vi "ep_Compute Third Current (Spectra).vi"(0 "complex current spectra in (5Hz step)":T2(array[cluster]), 5 "wiring":T3, 11 "error in (no error)":errorcluster) -> (4 "complex current spectra out (5Hz step)":T2(array[cluster]), 15 "error out":errorcluster)   [LabVIEW 2011, in "NI_EP_Power Quality.lvlib"]
uses:
  <vilib>/addons/Electrical Power/PQ/NI_EP_Power Quality.lvlib
  <vilib>/addons/Electrical Power/PQ/Common/Controls/ep_AI Data Channel.ctl
  <vilib>/addons/Electrical Power/PQ/Common/Controls/ep_Wiring.ctl
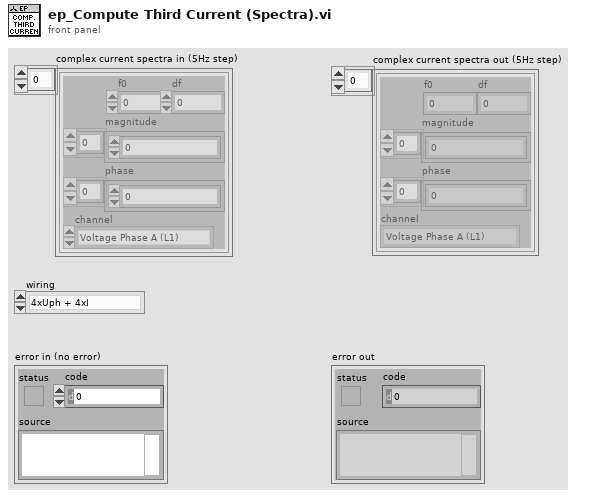
[diagram p1: front panel]
types:
  T1 = typedef "NI_EP_Power Quality.lvlib/ep_AI Data Channel.ctl" = enum16{"Voltage Phase A (L1)", "Voltage Phase B (L2)", "Voltage Phase C (L3)", "Voltage Phase N (Neutral)", "Current Phase A (L1)", "Current Phase B (L2)", "Current Phase C (L3)", "Current Phase N (Neutral)"}
  T2 = cluster{"f0":dbl, "df":dbl, "magnitude":dbl[], "phase":dbl[], "channel":T1}[]
  T3 = typedef "NI_EP_Power Quality.lvlib/ep_Wiring.ctl" = enum16{"4xUph + 4xI", "3xUph + 4xI", "3xUline + 4xI", "3xUph + 3xI", "3xUline + 3xI", "3xUph + 2xI", "3xUline + 2xI", "1xUph + 1xI"}
  T4 = cluster{"f0":dbl, "df":dbl, "magnitude":dbl[], "phase":dbl[], "channel":T1}
  T5 = cluster{"f0":dbl, "df":dbl, dbl[], dbl[], "AI data channel":T1}
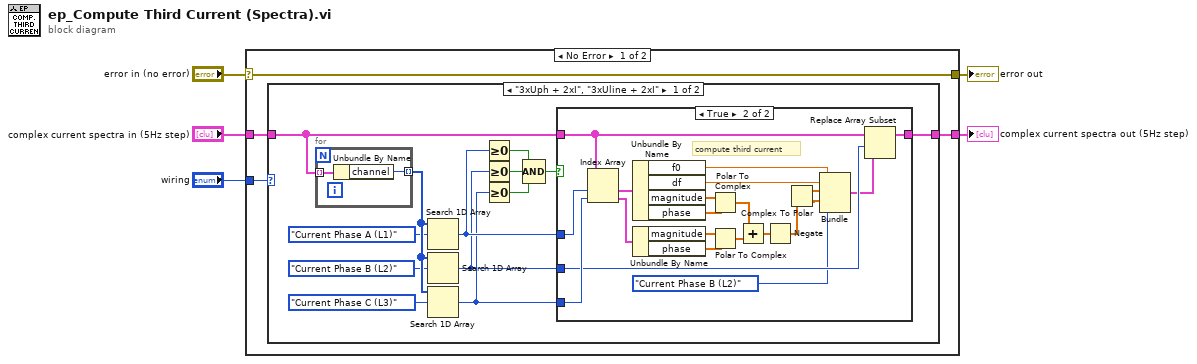
[diagram p0: block diagram]
diagram:
  n1 = case shown="No Error" "error in (no error)" {
    selector: "error in (no error)" -> [w6 w48]
    tunnel: "wiring" -> [w9 _]
    tunnel: [w8 _] -> w4
    tunnel: "complex current spectra in (5Hz step)" -> [w7 _]
    tunnel: [w6 w48] -> w1
    frame No Error {
      n2 = case shown="\"3xUph + 2xI\", \"3xUline + 2xI\"" w9 {
        tunnel: w7 -> [w11 w47]
        tunnel: [w22 w47] -> w8
        frame "3xUph + 2xI", "3xUline + 2xI" {
          n3 = for {
            tunnel: w11 -> [w46] mode=indexing
            tunnel: [w45] -> w19 mode=indexing
            n4 = Unbundle By Name(w46) -> ("channel"=w45:T1)
          }
          n5 = Search 1D Array(1D array=w19, element=ep_AI_Data_Channel."Current Phase A (L1)" ("AI data channel")) -> (index of element=w14:i32)  [unwired: 1 in]
          n6 = Search 1D Array(1D array=w19, element=ep_AI_Data_Channel."Current Phase B (L2)" ("AI data channel")) -> (index of element=w12:i32)  [unwired: 1 in]
          n7 = Search 1D Array(1D array=w19, element=ep_AI_Data_Channel."Current Phase C (L3)" ("AI data channel")) -> (index of element=w13:i32)  [unwired: 1 in]
          n8 = Greater Or Equal To 0?(x=w14) -> (x >= 0?=w10:bool)
          n9 = Greater Or Equal To 0?(x=w12) -> (x >= 0?=w20:bool)
          n10 = Greater Or Equal To 0?(x=w13) -> (x >= 0?=w21:bool)
          n11 = Compound Arithmetic op=AND(w10, w20, w21) -> (w15:bool)
          n12 = case shown="True" w15 {
            tunnel: [w23 w44] -> w22
            tunnel: w11 -> [w23 w43]
            tunnel: w14 -> [_ w42]
            tunnel: w13 -> [_ w41]
            tunnel: w12 -> [_ w40]
            frame False {
            }
            frame True {
              # "compute third current"
              n13 = Index Array(array=w43, index #1=w42, index #2=w41) -> (element #1=w39:T4, element #2=w38:T4)
              n14 = Unbundle By Name(w39) -> ("f0"=w36:dbl, "df"=w34:dbl, "magnitude"=w33:dbl[], "phase"=w32:dbl[])
              n15 = Unbundle By Name(w38) -> ("magnitude"=w30:dbl[], "phase"=w29:dbl[])
              n16 = Polar To Complex(1:w32, 2:w33) -> (0:w31:cdb[])
              n17 = Polar To Complex(1:w29, 2:w30) -> (0:w28:cdb[])
              n18 = Add(x=w31, y=w28) -> (x+y=w37:cdb[])
              n19 = Negate(x=w37) -> (-x=w24:cdb[])
              n20 = Complex To Polar(r * e^(i*theta)=w24) -> (r=w26:dbl[], theta=w25:dbl[])
              n21 = Bundle("f0"=w36, "df"=w34, w26, w25, "AI data channel"=ep_AI_Data_Channel."Current Phase B (L2)") -> (w35:T5)  [unwired: 1 in]
              n22 = Replace Array Subset(array=w43, new element=w35, index=w40) -> (w44:T2)
            }
          }
        }
        frame Default {
        }
      }
    }
    frame Error {
    }
  }
  "error out" <- w1
  "complex current spectra out (5Hz step)" <- w4
